vi "Finish.vi"(4 "error in":errorcluster) -> ()   [LabVIEW 2013]
doc: "This VI is called just before exiting. It is expected to close I/O refnum, save collected data, etc."
uses:
  <vilib>/Rock Robotics/WPI/Solenoid/WPI_SolenoidValue.ctl
  <vilib>/Rock Robotics/WPI/RobotDrive/WPI_RobotDriveGetSetRefNum.vi
  <vilib>/Rock Robotics/WPI/Joystick/WPI_JoystickGetSetRefNum.vi
  <vilib>/Rock Robotics/WPI/Solenoid/WPI_SolenoidSetEnum.vi
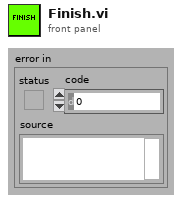
[diagram p1: front panel]
types:
  T1 = typedef "WPI_DigitalInputDevRef.ctl" = cluster{"DevStatus":errorcluster, "DIO Channel":T2, "Digital Module":T3}
  T2 = typedef "FPGA_DIOChannel.ctl" = enum8{"DIO 1", "DIO 2", "DIO 3", "DIO 4", "DIO 5", "DIO 6", "DIO 7", "DIO 8", "DIO 9", "DIO 10", "DIO 11", "DIO 12", "DIO 13", "DIO 14", "Invalid"}
  T3 = typedef "FPGA_TypedefDigitalModule.ctl" = enum16{"Digital Module 1", "Digital Module 2"}
  T4 = typedef "WPI_JoystickDevRef.ctl" = cluster{"Device":T5}
  T5 = typedef "WPI_JoystickDeviceEnum.ctl" = enum16{"USB 1", "USB 2", "USB 3", "USB 4", "Kinect 1", "Kinect 2"}
  T6 = typedef "WPI_CameraDevRef.ctl" = cluster{"Camera Address":string, "CameraStatus":errorcluster, "Acquire Image Notifier":refnum<notifier>}
  T7 = typedef "WPI_RobotDriveDevRef.ctl" = cluster{"DevStatus":errorcluster, "Motors[]":T8[], "Square Inputs":bool, "Max Output":dbl, "Isochronous":bool}
  T8 = typedef "WPI_MotorControlDeviceRef.ctl" = cluster{"DeviceStatus":errorcluster, "Type":enum16{"PWM", "CAN"}, "PWM":cluster{"Digital Module":T3, "PWM Channel":T9, "DeadBand":T10}, "CAN":cluster{"Device Number":u8, "Control Mode":T11, "Semaphore":T12, "Max Vout":dbl}, "Invert":bool, "TransformRef":T13, "InvTransformRef":T13}
  T9 = typedef "FPGA_DIOPWMChannel.ctl" = enum8{"PWM 1", "PWM 2", "PWM 3", "PWM 4", "PWM 5", "PWM 6", "PWM 7", "PWM 8", "PWM 9", "PWM 10", "Invalid"}
  T10 = typedef "WPI_PWMDeadband.ctl" = cluster{"Name":string, "maxPositivePwm":i32, "minPositivePwm":i32, "centerPwm":i32, "maxNegativePwm":i32, "minNegativePwm":i32, "angularRange":u16}
  T11 = typedef "WPI_CANJaguar_ControlMode.ctl" = enum8{"Percent VBus", "Current", "Speed", "Position", "Voltage"}
  T12 = typedef "Semaphore RefNum" = refnum<k1>
  T13 = typedef "WPI_PWMTransform_ConPane.ctl" = refnum<vi>
  T14 = typedef "WPI_EncoderDevRef.ctl" = cluster{"DevStatus":errorcluster, "EncoderIndex":T15, "CounterIndex":T16, "DistancePerCount":dbl, "Decoding Type":T17}
  T15 = typedef "FPGA_EncoderIdx.ctl" = enum8{"Enc 0", "Enc 1", "Enc 2", "Enc 3", "Invalid"}
  T16 = typedef "FPGA_CounterCtrSystemIndex.ctl" = enum8{"Ctr 0", "Ctr 1", "Ctr 2", "Ctr 3", "Ctr 4", "Ctr 5", "Ctr 6", "Ctr 7", "Invalid"}
  T17 = typedef "WPI_EncoderType.ctl" = enum16{"1x", "2x", "4x"}
  T18 = typedef "WPI_SolenoidDevRef.ctl" = cluster{"DevStatus":errorcluster, "Solenoid Module":T19, "Forward Solenoid Channel":T20, "Reverse Solenoid Channel":T20}
  T19 = typedef "FPGA_TypedefSolenoidModule.ctl" = enum16{"Solenoid Module 1", "Solenoid Module 2"}
  T20 = typedef "WPI_SolenoidChannel.ctl" = enum8{"Solenoid 1", "Solenoid 2", "Solenoid 3", "Solenoid 4", "Solenoid 5", "Solenoid 6", "Solenoid 7", "Solenoid 8", "Invalid"}
  T21 = typedef "WPI_SolenoidValue.ctl" = enum16{"Off", "On", "Forward", "Reverse"}
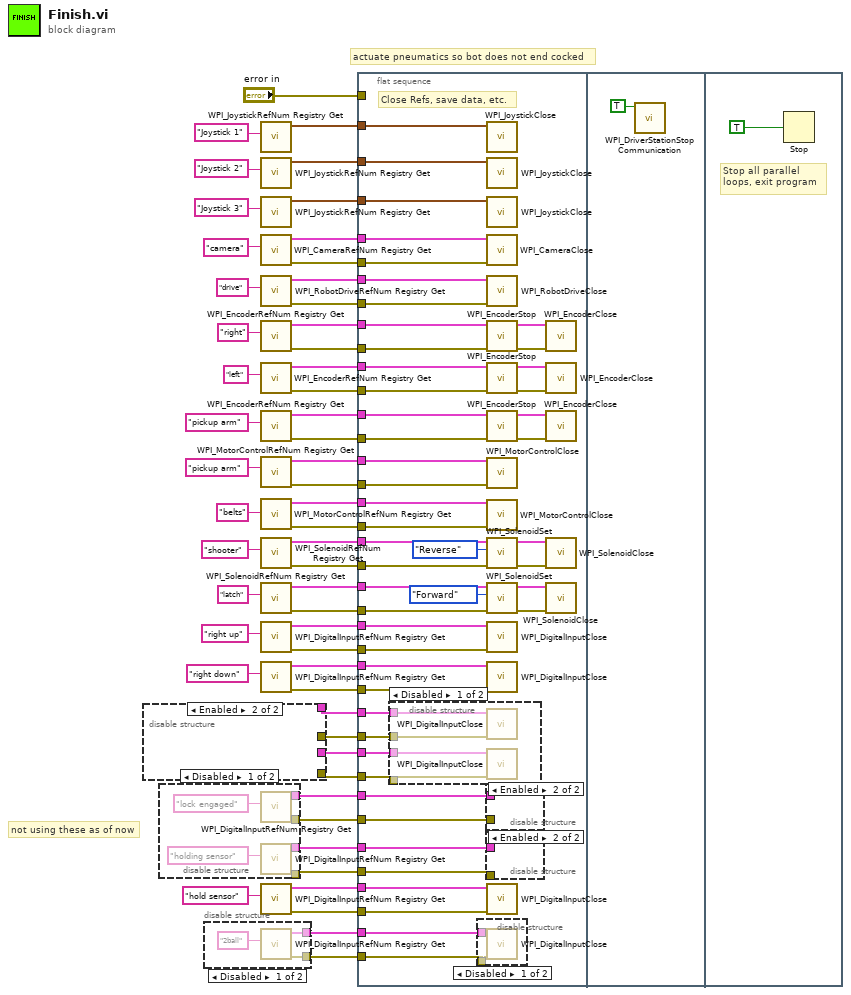
[diagram p0: block diagram]
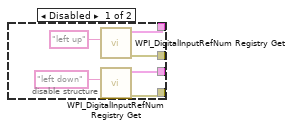
[diagram p3: hidden frame]
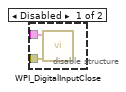
[diagram p7: hidden frame]
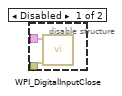
[diagram p8: hidden frame]
diagram:
  # "not using these as of now"
  # "actuate pneumatics so bot does not end cocked"
  n1 = disable-structure shown="Enabled" {
    disable-tunnel: [w57 _] -> w13
    disable-tunnel: [w56 _] -> w12
    disable-tunnel: [w55 _] -> w11
    disable-tunnel: [w54 _] -> w10
    frame Disabled {
      n2 = call <vilib>:"WPI_DigitalInputRefNum Registry Get.vi"("refnum name"="left up") -> ("error out"=w56:errorcluster, "DigitalInputDevRef"=w57:T1)  [unwired: 9 in]
      n3 = call <vilib>:"WPI_DigitalInputRefNum Registry Get.vi"("refnum name"="left down") -> ("error out"=w54:errorcluster, "DigitalInputDevRef"=w55:T1)  [unwired: 9 in]
    }
    frame Enabled {
    }
  }
  n4 = disable-structure shown="Disabled" {
    disable-tunnel: [w65 _] -> w7
    disable-tunnel: [w64 _] -> w6
    disable-tunnel: [w62 _] -> w4
    disable-tunnel: [w61 _] -> w3
    frame Disabled {
      n5 = call <vilib>:"WPI_DigitalInputRefNum Registry Get.vi"("refnum name"="lock engaged") -> ("error out"=w62:errorcluster, "DigitalInputDevRef"=w61:T1)  [unwired: 9 in]
      n6 = call <vilib>:"WPI_DigitalInputRefNum Registry Get.vi"("refnum name"="holding sensor") -> ("error out"=w65:errorcluster, "DigitalInputDevRef"=w64:T1)  [unwired: 9 in]
    }
    frame Enabled {
    }
  }
  n7 = disable-structure shown="Disabled" {
    disable-tunnel: [w67 _] -> w2
    disable-tunnel: [w66 _] -> w1
    frame Disabled {
      n8 = call <vilib>:"WPI_DigitalInputRefNum Registry Get.vi"("refnum name"="2ball") -> ("error out"=w66:errorcluster, "DigitalInputDevRef"=w67:T1)  [unwired: 9 in]
    }
    frame Enabled {
    }
  }
  n9 = call <vilib>:"WPI_JoystickRefNum Registry Get.vi"("refnum name"="Joystick 1") -> ("JoystickDevRef"=w52:T4)  [unwired: 1 in, 9 out]
  n10 = call <vilib>:"WPI_JoystickRefNum Registry Get.vi"("refnum name"="Joystick 2") -> ("JoystickDevRef"=w49:T4)  [unwired: 1 in, 9 out]
  n11 = call <vilib>:"WPI_JoystickRefNum Registry Get.vi"("refnum name"="Joystick 3") -> ("JoystickDevRef"=w46:T4)  [unwired: 1 in, 9 out]
  n12 = call <vilib>:"WPI_CameraRefNum Registry Get.vi"("refnum name"="camera") -> ("error out"=w39:errorcluster, "CameraDevRef"=w51:T6)  [unwired: 1 in, 8 out]
  n13 = call <vilib>:"WPI_RobotDriveRefNum Registry Get.vi"("refnum name"="drive") -> ("error out"=w38:errorcluster, "RobotDriveDevRef"=w44:T7)  [unwired: 9 in]
  n14 = call <vilib>:"WPI_EncoderRefNum Registry Get.vi"("refnum name"="right") -> ("error out"=w37:errorcluster, "EncoderDevRef"=w41:T14)  [unwired: 9 in]
  n15 = call <vilib>:"WPI_EncoderRefNum Registry Get.vi"("refnum name"="left") -> ("error out"=w36:errorcluster, "EncoderDevRef"=w40:T14)  [unwired: 9 in]
  n16 = call <vilib>:"WPI_EncoderRefNum Registry Get.vi"("refnum name"="pickup arm") -> ("error out"=w35:errorcluster, "EncoderDevRef"=w33:T14)  [unwired: 9 in]
  n17 = call <vilib>:"WPI_MotorControlRefNum Registry Get.vi"("refnum name"="pickup arm") -> ("error out"=w29:errorcluster, "MotorControlDevRef"=w30:T8)  [unwired: 9 in]
  n18 = call <vilib>:"WPI_MotorControlRefNum Registry Get.vi"("refnum name"="belts") -> ("error out"=w27:errorcluster, "MotorControlDevRef"=w28:T8)  [unwired: 9 in]
  n19 = call <vilib>:"WPI_SolenoidRefNum Registry Get.vi"("refnum name"="shooter") -> ("error out"=w25:errorcluster, "SolenoidDevRef"=w26:T18)  [unwired: 9 in]
  n20 = call <vilib>:"WPI_SolenoidRefNum Registry Get.vi"("refnum name"="latch") -> ("error out"=w21:errorcluster, "SolenoidDevRef"=w22:T18)  [unwired: 9 in]
  n21 = call <vilib>:"WPI_DigitalInputRefNum Registry Get.vi"("refnum name"="right up") -> ("error out"=w16:errorcluster, "DigitalInputDevRef"=w17:T1)  [unwired: 9 in]
  n22 = call <vilib>:"WPI_DigitalInputRefNum Registry Get.vi"("refnum name"="right down") -> ("error out"=w14:errorcluster, "DigitalInputDevRef"=w15:T1)  [unwired: 9 in]
  n23 = call <vilib>:"WPI_DigitalInputRefNum Registry Get.vi"("refnum name"="hold sensor") -> ("error out"=w9:errorcluster, "DigitalInputDevRef"=w8:T1)  [unwired: 9 in]
  n24 = flat-sequence {
    tunnel: w52 -> [w117]
    tunnel: w51 -> [w116]
    tunnel: w49 -> [w115]
    tunnel: w46 -> [w114]
    tunnel: w44 -> [w113]
    tunnel: w41 -> [w112]
    tunnel: w40 -> [w105]
    tunnel: w39 -> [w109]
    tunnel: w38 -> [w108]
    tunnel: w37 -> [w107]
    tunnel: w36 -> [w106]
    tunnel: w35 -> [w101]
    tunnel: w33 -> [w100]
    tunnel: w30 -> [w98]
    tunnel: w29 -> [w97]
    tunnel: w28 -> [w95]
    tunnel: w27 -> [w96]
    tunnel: w26 -> [w78]
    tunnel: w25 -> [w77]
    tunnel: w22 -> [w74]
    tunnel: w21 -> [w73]
    tunnel: "error in" -> [_]
    tunnel: w17 -> [w90]
    tunnel: w16 -> [w91]
    tunnel: w15 -> [w89]
    tunnel: w14 -> [w92]
    tunnel: w13 -> [w88]
    tunnel: w12 -> [w93]
    tunnel: w11 -> [w87]
    tunnel: w10 -> [w94]
    tunnel: w6 -> [w85]
    tunnel: w7 -> [w84]
    tunnel: w8 -> [w86]
    tunnel: w9 -> [w83]
    tunnel: w3 -> [w82]
    tunnel: w4 -> [w81]
    tunnel: w2 -> [w79]
    tunnel: w1 -> [w80]
    frame #0 {
      # "Close Refs, save data, etc."
      n25 = disable-structure shown="Disabled" {
        disable-tunnel: w94 -> [w123 _]
        disable-tunnel: w93 -> [w122 _]
        disable-tunnel: w88 -> [w121 _]
        disable-tunnel: w87 -> [w120 _]
        frame Disabled {
          n26 = call <vilib>:"WPI_DigitalInputClose.vi"("error in (no error)"=w122, "DigitalInputDevRef"=w121) -> ()  [unwired: 9 in, 1 out]
          n27 = call <vilib>:"WPI_DigitalInputClose.vi"("error in (no error)"=w123, "DigitalInputDevRef"=w120) -> ()  [unwired: 9 in, 1 out]
        }
        frame Enabled {
        }
      }
      n28 = disable-structure shown="Disabled" {
        disable-tunnel: w80 -> [w119 _]
        disable-tunnel: w79 -> [w118 _]
        frame Disabled {
          n29 = call <vilib>:"WPI_DigitalInputClose.vi"("error in (no error)"=w119, "DigitalInputDevRef"=w118) -> ()  [unwired: 9 in, 1 out]
        }
        frame Enabled {
        }
      }
      n30 = call <vilib>:"WPI_JoystickClose.vi"("JoystickDevRef"=w117) -> ()  [unwired: 11 out]
      n31 = call <vilib>:"WPI_JoystickClose.vi"("JoystickDevRef"=w115) -> ()  [unwired: 11 out]
      n32 = call <vilib>:"WPI_JoystickClose.vi"("JoystickDevRef"=w114) -> ()  [unwired: 11 out]
      n33 = call <vilib>:"WPI_CameraClose.vi"("error in (no error)"=w109, "CameraDevRef"=w116) -> ()  [unwired: 10 out]
      n34 = call <vilib>:"WPI_RobotDriveClose.vi"("error in (no error)"=w108, "RobotDriveDevRef"=w113) -> ()  [unwired: 9 in, 1 out]
      n35 = call <vilib>:"WPI_EncoderStop.vi"("error in (no error)"=w107, "EncoderDevRef"=w112) -> ("error out"=w111:errorcluster, "EncoderDevRef"=w110:T14)  [unwired: 8 in]
      n36 = call <vilib>:"WPI_EncoderStop.vi"("error in (no error)"=w106, "EncoderDevRef"=w105) -> ("error out"=w103:errorcluster, "EncoderDevRef"=w104:T14)  [unwired: 8 in]
      n37 = call <vilib>:"WPI_EncoderStop.vi"("error in (no error)"=w101, "EncoderDevRef"=w100) -> ("error out"=w102:errorcluster, "EncoderDevRef"=w99:T14)  [unwired: 8 in]
      n38 = call <vilib>:"WPI_MotorControlClose.vi"("error in (no error)"=w97, "MotorControlDevRef"=w98) -> ()  [unwired: 9 in, 1 out]
      n39 = call <vilib>:"WPI_MotorControlClose.vi"("error in (no error)"=w96, "MotorControlDevRef"=w95) -> ()  [unwired: 9 in, 1 out]
      n40 = call-poly <vilib>:"WPI_SolenoidSet.vi"("error in (no error)"=w77, "Value"=WPI_SolenoidValue."Reverse", "SolenoidDevRef"=w78) -> ("error out"=w70:errorcluster, "SolenoidDevRef"=w69:T18)  [unwired: 7 in]
      n41 = call-poly <vilib>:"WPI_SolenoidSet.vi"("error in (no error)"=w73, "Value"=WPI_SolenoidValue."Forward", "SolenoidDevRef"=w74) -> ("error out"=w76:errorcluster, "SolenoidDevRef"=w75:T18)  [unwired: 7 in]
      n42 = call <vilib>:"WPI_DigitalInputClose.vi"("error in (no error)"=w91, "DigitalInputDevRef"=w90) -> ()  [unwired: 9 in, 1 out]
      n43 = call <vilib>:"WPI_DigitalInputClose.vi"("error in (no error)"=w92, "DigitalInputDevRef"=w89) -> ()  [unwired: 9 in, 1 out]
      n44 = disable-structure shown="Enabled" {
        disable-tunnel: w82 -> [w125 _]
        disable-tunnel: w81 -> [w124 _]
        frame Disabled {
          n45 = call <vilib>:"WPI_DigitalInputClose.vi"("error in (no error)"=w124, "DigitalInputDevRef"=w125) -> ()  [unwired: 9 in, 1 out]
        }
        frame Enabled {
        }
      }
      n46 = disable-structure shown="Enabled" {
        disable-tunnel: w85 -> [w127 _]
        disable-tunnel: w84 -> [w126 _]
        frame Disabled {
          n47 = call <vilib>:"WPI_DigitalInputClose.vi"("error in (no error)"=w126, "DigitalInputDevRef"=w127) -> ()  [unwired: 9 in, 1 out]
        }
        frame Enabled {
        }
      }
      n48 = call <vilib>:"WPI_DigitalInputClose.vi"("error in (no error)"=w83, "DigitalInputDevRef"=w86) -> ()  [unwired: 9 in, 1 out]
      n49 = call <vilib>:"WPI_EncoderClose.vi"("error in (no error)"=w111, "EncoderDevRef"=w110) -> ()  [unwired: 9 in, 1 out]
      n50 = call <vilib>:"WPI_EncoderClose.vi"("error in (no error)"=w103, "EncoderDevRef"=w104) -> ()  [unwired: 9 in, 1 out]
      n51 = call <vilib>:"WPI_EncoderClose.vi"("error in (no error)"=w102, "EncoderDevRef"=w99) -> ()  [unwired: 9 in, 1 out]
      n52 = call <vilib>:"WPI_SolenoidClose.vi"("error in (no error)"=w70, "SolenoidDevRef"=w69) -> ()  [unwired: 9 in, 1 out]
      n53 = call <vilib>:"WPI_SolenoidClose.vi"("error in (no error)"=w76, "SolenoidDevRef"=w75) -> ()  [unwired: 9 in, 1 out]
    }
    frame #1 {
      n54 = call <vilib>:"WPI_DriverStationStop Communication.vi"("StopCommunication"=TRUE) -> ()  [unwired: 10 in, 1 out]
    }
    frame #2 {
      # "Stop all parallel\nloops, exit program"
      n55 = Stop(stop? (T)=TRUE ("Quit")) -> ()
    }
  }
